vi "CmdCluster2ParameterSet.vi"(0 "CMDCluster":T1, 7 "Controller?":bool) -> (4 "ParameterSet":string)   [LabVIEW 2013]
uses:
  TypeDef/Command Cluster.ctl
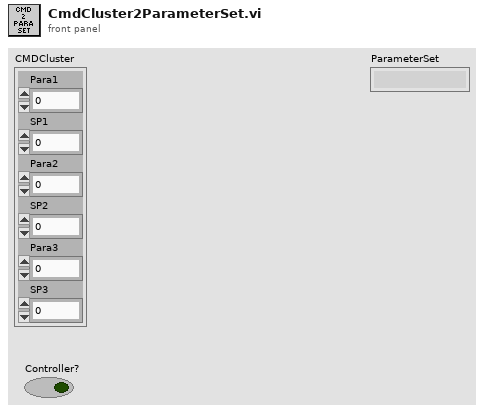
[diagram p1: front panel]
types:
  T1 = typedef "Command Cluster.ctl" = cluster{"Para1":i32, "SP1":dbl, "Para2":i32, "SP2":dbl, "Para3":i32, "SP3":dbl}
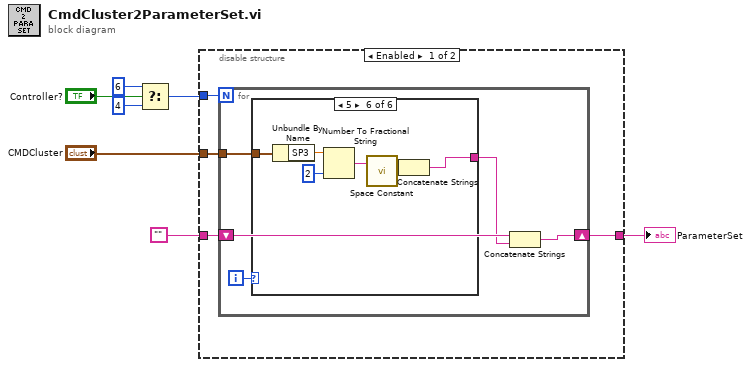
[diagram p0: block diagram]
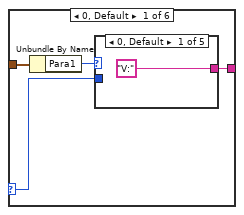
[diagram p2: hidden frame]
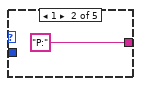
[diagram p3: hidden frame]
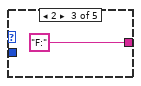
[diagram p4: hidden frame]
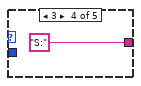
[diagram p5: hidden frame]
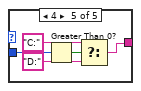
[diagram p6: hidden frame]
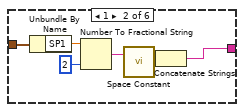
[diagram p7: hidden frame]
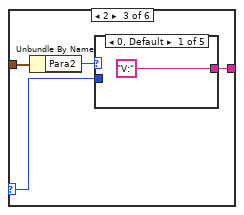
[diagram p8: hidden frame]
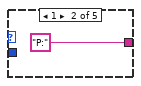
[diagram p9: hidden frame]
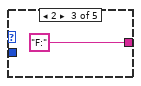
[diagram p10: hidden frame]
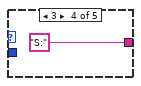
[diagram p11: hidden frame]
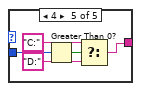
[diagram p12: hidden frame]
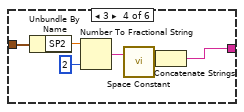
[diagram p13: hidden frame]
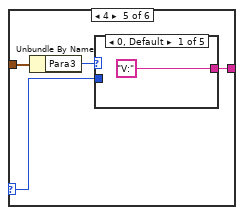
[diagram p14: hidden frame]
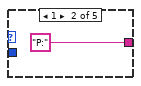
[diagram p15: hidden frame]
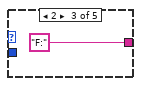
[diagram p16: hidden frame]
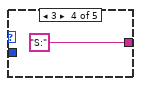
[diagram p17: hidden frame]
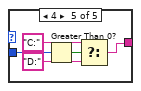
[diagram p18: hidden frame]
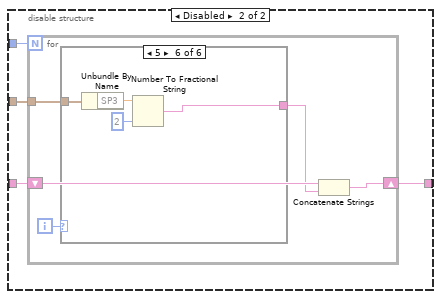
[diagram p19: hidden frame]
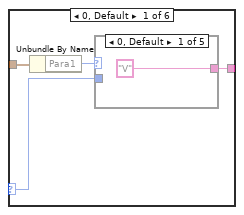
[diagram p20: hidden frame]
diagram:
  n1 = Select(t=6, s="Controller?", f=4) -> (s? t:f=w4:i32)
  n2 = disable-structure shown="Enabled" {
    disable-tunnel: "CMDCluster" -> [w11 w77]
    disable-tunnel: "" -> [w10 w76]
    disable-tunnel: w4 -> [w9 w75]
    disable-tunnel: [w8 w74] -> w1
    frame Enabled {
      n3 = for {
        N: w9 -> [_]
        tunnel: w11 -> [w15]
        shift-right: [w12] -> w8
        shift-left: w10 -> [w14]
        i -> [w16]
        n4 = case shown="5" w16 {
          selector: w16 -> [w18 _ w36 _ w55 _]
          tunnel: w15 -> [w20 w35 w39 w54 w58 w73]
          tunnel: [w17 w30 w37 w49 w56 w68] -> w13
          frame 0, Default {
            n5 = Unbundle By Name(w20) -> ("Para1"=w19:i32)
            n6 = case shown="0, Default" w19 {
              tunnel: ["V:" "P:" "F:" "S:" w25] -> w17
              tunnel: w18 -> [_ _ _ _ w29]
              frame 0, Default {
              }
              frame 1 {
              }
              frame 2 {
              }
              frame 3 {
              }
              frame 4 {
                n7 = Greater Than 0?(x=w29) -> (x > 0?=w28:bool)
                n8 = Select(t="C:", s=w28, f="D:") -> (s? t:f=w25:string)
              }
            }
          }
          frame 1 {
            n9 = Unbundle By Name(w35) -> ("SP1"=w34:dbl)
            n10 = Number To Fractional String(number=w34, precision (6)=i16 2) -> (F-format string=w32:string)  [unwired: 2 in]
            n11 = call <vilib>:"Space Constant.vi"() -> ("String"=w31:string)
            n12 = Concatenate Strings(w32, w31) -> (w30:string)
          }
          frame 2 {
            n13 = Unbundle By Name(w39) -> ("Para2"=w38:i32)
            n14 = case shown="0, Default" w38 {
              tunnel: ["V:" "P:" "F:" "S:" w44] -> w37
              tunnel: w36 -> [_ _ _ _ w48]
              frame 0, Default {
              }
              frame 1 {
              }
              frame 2 {
              }
              frame 3 {
              }
              frame 4 {
                n15 = Greater Than 0?(x=w48) -> (x > 0?=w47:bool)
                n16 = Select(t="C:", s=w47, f="D:") -> (s? t:f=w44:string)
              }
            }
          }
          frame 3 {
            n17 = Unbundle By Name(w54) -> ("SP2"=w52:dbl)
            n18 = Number To Fractional String(number=w52, precision (6)=i16 2) -> (F-format string=w50:string)  [unwired: 2 in]
            n19 = call <vilib>:"Space Constant.vi"() -> ("String"=w51:string)
            n20 = Concatenate Strings(w50, w51) -> (w49:string)
          }
          frame 4 {
            n21 = Unbundle By Name(w58) -> ("Para3"=w57:i32)
            n22 = case shown="0, Default" w57 {
              tunnel: ["V:" "P:" "F:" "S:" w63] -> w56
              tunnel: w55 -> [_ _ _ _ w67]
              frame 0, Default {
              }
              frame 1 {
              }
              frame 2 {
              }
              frame 3 {
              }
              frame 4 {
                n23 = Greater Than 0?(x=w67) -> (x > 0?=w66:bool)
                n24 = Select(t="C:", s=w66, f="D:") -> (s? t:f=w63:string)
              }
            }
          }
          frame 5 {
            n25 = Unbundle By Name(w73) -> ("SP3"=w71:dbl)
            n26 = Number To Fractional String(number=w71, precision (6)=i16 2) -> (F-format string=w69:string)  [unwired: 2 in]
            n27 = call <vilib>:"Space Constant.vi"() -> ("String"=w70:string)
            n28 = Concatenate Strings(w69, w70) -> (w68:string)
          }
        }
        n29 = Concatenate Strings(w14, w13) -> (w12:string)
      }
    }
    frame Disabled {
      n30 = for {
        N: w75 -> [_]
        tunnel: w77 -> [w81]
        shift-right: [w78] -> w74
        shift-left: w76 -> [w80]
        i -> [w82]
        n31 = case shown="5" w82 {
          selector: w82 -> [w84 _ w100 _ w117 _]
          tunnel: w81 -> [w86 w99 w103 w116 w120 w133]
          tunnel: [w83 w96 w101 w113 w118 w130] -> w79
          frame 0, Default {
            n32 = Unbundle By Name(w86) -> ("Para1"=w85:i32)
            n33 = case shown="0, Default" w85 {
              tunnel: ["V" "P" "F" "S" w91] -> w83
              tunnel: w84 -> [_ _ _ _ w95]
              frame 0, Default {
              }
              frame 1 {
              }
              frame 2 {
              }
              frame 3 {
              }
              frame 4 {
                n34 = Greater Than 0?(x=w95) -> (x > 0?=w94:bool)
                n35 = Select(t="C", s=w94, f="D") -> (s? t:f=w91:string)
              }
            }
          }
          frame 1 {
            n36 = Unbundle By Name(w99) -> ("SP1"=w98:dbl)
            n37 = Number To Fractional String(number=w98, precision (6)=i16 2) -> (F-format string=w96:string)  [unwired: 2 in]
          }
          frame 2 {
            n38 = Unbundle By Name(w103) -> ("Para2"=w102:i32)
            n39 = case shown="0, Default" w102 {
              tunnel: ["V" "P" "F" "S" w108] -> w101
              tunnel: w100 -> [_ _ _ _ w112]
              frame 0, Default {
              }
              frame 1 {
              }
              frame 2 {
              }
              frame 3 {
              }
              frame 4 {
                n40 = Greater Than 0?(x=w112) -> (x > 0?=w111:bool)
                n41 = Select(t="C", s=w111, f="D") -> (s? t:f=w108:string)
              }
            }
          }
          frame 3 {
            n42 = Unbundle By Name(w116) -> ("SP2"=w114:dbl)
            n43 = Number To Fractional String(number=w114, precision (6)=i16 2) -> (F-format string=w113:string)  [unwired: 2 in]
          }
          frame 4 {
            n44 = Unbundle By Name(w120) -> ("Para3"=w119:i32)
            n45 = case shown="0, Default" w119 {
              tunnel: ["V" "P" "F" "S" w125] -> w118
              tunnel: w117 -> [_ _ _ _ w129]
              frame 0, Default {
              }
              frame 1 {
              }
              frame 2 {
              }
              frame 3 {
              }
              frame 4 {
                n46 = Greater Than 0?(x=w129) -> (x > 0?=w128:bool)
                n47 = Select(t="C", s=w128, f="D") -> (s? t:f=w125:string)
              }
            }
          }
          frame 5 {
            n48 = Unbundle By Name(w133) -> ("SP3"=w131:dbl)
            n49 = Number To Fractional String(number=w131, precision (6)=i16 2) -> (F-format string=w130:string)  [unwired: 2 in]
          }
        }
        n50 = Concatenate Strings(w80, w79) -> (w78:string)
      }
    }
  }
  "ParameterSet" <- w1
